vi "Set Class Color.vi"(8 "error in (no error)":errorcluster, 9 "Element Type":variant, 11 "LVLibrary in":refnum<vi>) -> (0 "error out":errorcluster, 3 "LVLibrary out":refnum<vi>)   [LabVIEW 2020, in "FlexBlocks.lvlib"]
uses:
  FlexBlocks.lvlib
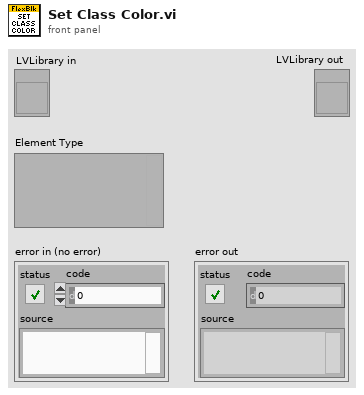
[diagram p1: front panel]
types:
  T1 = cluster{"Foreground Color":u32, "Background Color":u32, "Fill Pattern":cluster{"Row 0":u8, "Row 1":u8, "Row 2":u8, "Row 3":u8, "Row 4":u8, "Row 5":u8, "Row 6":u8, "Row 7":u8}, "Width":i16, "Mode":enum16{"Copy", "Or", "Exclusive Or", "Bit Clear", "Not Copy", "Not Or", "Nor Exclusive Or", "Not Bit Clear"}, "Style":enum32{"Solid", "Dash", "Dot", "Dash Dot", "Dash Dot Dot"}, "Fill Rule":enum32{"Even Odd", "Winding"}, "End Caps":enum32{"Default", "Flat"}}[]
  T2 = cluster{"Foreground Color":u32, "Background Color":u32, "Fill Pattern":cluster{"Row 0":u8, "Row 1":u8, "Row 2":u8, "Row 3":u8, "Row 4":u8, "Row 5":u8, "Row 6":u8, "Row 7":u8}, "Width":i16, "Mode":enum16{"Copy", "Or", "Exclusive Or", "Bit Clear", "Not Copy", "Not Or", "Nor Exclusive Or", "Not Bit Clear"}, "Style":enum32{"Solid", "Dash", "Dot", "Dash Dot", "Dash Dot Dot"}, "Fill Rule":enum32{"Even Odd", "Winding"}, "End Caps":enum32{"Default", "Flat"}}
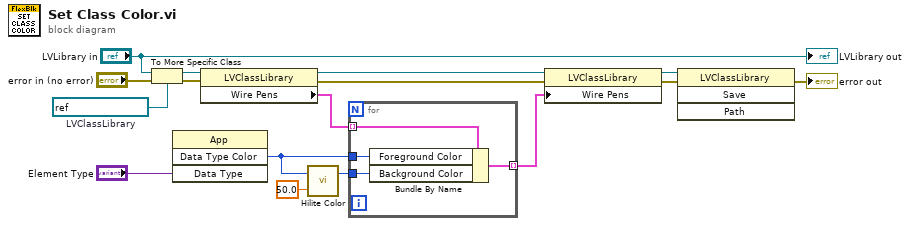
[diagram p0: block diagram]
diagram:
  w16 = refnum<vi> refnum  # LVClassLibrary
  n1 = To More Specific Class(target class=w16, reference="LVLibrary in", error in="error in (no error)") -> (specific class reference=w15:refnum<vi>, error out=w6:errorcluster)
  n2 = invoke class="App" method="Data Type Color"("Data Type"="Element Type") -> ("Data Type Color"=w9:u32)  [unwired: 3 in, 3 out]
  n3 = property class="LVClassLibrary"(reference=w15, error in=w6) -> (reference out=w8:refnum<vi>, error out=w5:errorcluster, "Wire Pens"=w11:T1)
  n4 = call <vilib>:"Hilite Color.vi"("Percentage(30)"=50.0, "Color In"=w9) -> ("Hilite"=w10:u32)  [unwired: 1 out]
  n5 = for {
    tunnel: w11 -> [w20] mode=indexing
    tunnel: w10 -> [w18]
    tunnel: w9 -> [w19]
    tunnel: [w17] -> w7 mode=indexing
    n6 = Bundle By Name(cluster=w20, "Foreground Color"=w19, "Background Color"=w18) -> (w17:T2)
  }
  n7 = property class="LVClassLibrary"(reference=w8, error in=w5, "Wire Pens"=w7) -> (reference out=w4:refnum<vi>, error out=w3:errorcluster)
  n8 = invoke class="LVClassLibrary" method="Save"(reference=w4, error in=w3) -> (error out=→"error out":errorcluster)  [unwired: 2 in, 3 out]
  "LVLibrary out" <- "LVLibrary in"
